vi "ControlGuiWindow.vi"(8 "error in (no error)":errorcluster, 10 "ShowProcessWindow":bool, 11 "reference in":refnum<class "RemoteControl.lvclass">) -> (0 "error out":errorcluster, 3 "reference out":refnum<class "RemoteControl.lvclass">)   [LabVIEW 2020, in "RemoteControl.lvclass"]
uses:
  RemoteControl.lvclass
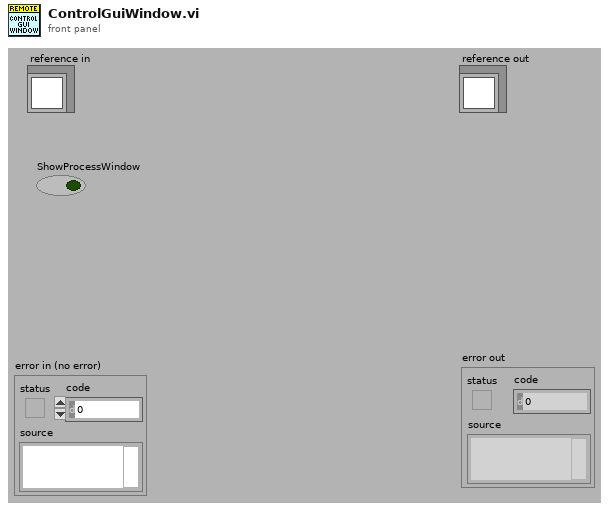
[diagram p1: front panel]
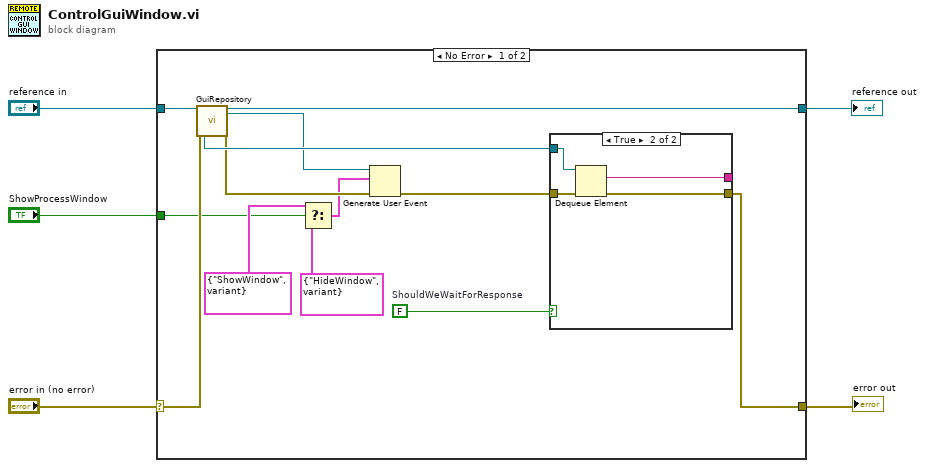
[diagram p0: block diagram]
diagram:
  n1 = case shown="No Error" "error in (no error)" {
    selector: "error in (no error)" -> [w18 w25]
    tunnel: [w10 w25] -> w4
    tunnel: [w16 w24] -> w2
    tunnel: "reference in" -> [w17 w24]
    tunnel: "ShowProcessWindow" -> [w7 _]
    frame No Error {
      w15 = FALSE  # ShouldWeWaitForResponse
      n2 = call "GuiRepository.vi"("reference in"=w17, "error in (no error)"=w18) -> ("QueueFromProcess"=w13:refnum<queue>, "reference out"=w16:refnum<class "RemoteControl.lvclass">, "EventsToProcess"=w11:refnum<user-event>, "error out"=w12:errorcluster)  [unwired: 10 in, 4 out]
      n3 = Select(t=cluster{"Command":string, "Data":variant} {"Command"="ShowWindow", "Data"=variant} ("MessageToProcess"), s=w7, f=cluster{"Command":string, "Data":variant} {"Command"="HideWindow", "Data"=variant} ("MessageToProcess")) -> (s? t:f=w6:cluster{"Command":string, "Data":variant})
      n4 = Generate User Event(user event=w11, event data cluster=w6, error in=w12) -> (error out=w14:errorcluster)  [unwired: 1 in, 1 out]
      n5 = case shown="True" w15 {
        tunnel: w14 -> [w19 w23]
        tunnel: w13 -> [_ w22]
        tunnel: [_ w21] -> _
        tunnel: [w19 w20] -> w10
        frame False {
        }
        frame True {
          n6 = Dequeue Element(queue=w22, error in (no error)=w23) -> (element=w21:string, error out=w20:errorcluster)  [unwired: 1 in, 2 out]
        }
      }
    }
    frame Error {
    }
  }
  "error out" <- w4
  "reference out" <- w2
